vi "Get Sub Object.vi"(8 "error in":errorcluster, 9 "Sub Index":u8 format="%02x", 10 "Index":u16 format="%04x", 11 "Obj Dict in":refnum<class "Object Dictionary.lvclass">) -> (0 "error out":errorcluster, 2 "Sub Obj":refnum<class "Sub Object.lvclass">, 3 "Obj Dict out":refnum<class "Object Dictionary.lvclass">)   [LabVIEW 2020, in "CANopen.lvlib" / "Object Dictionary.lvclass"]
uses:
  Object Dictionary.lvclass
  Sub Object/Sub Object.lvclass
  Object Entry/Object Entry.lvclass
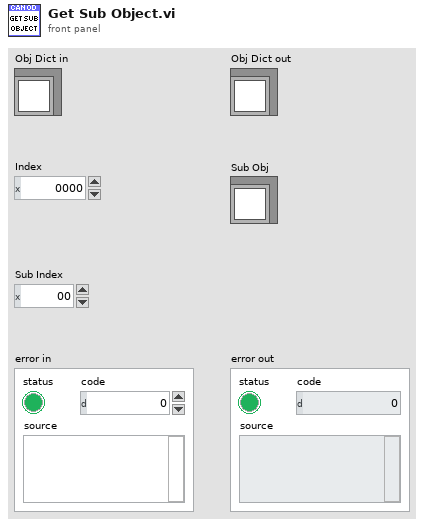
[diagram p1: front panel]
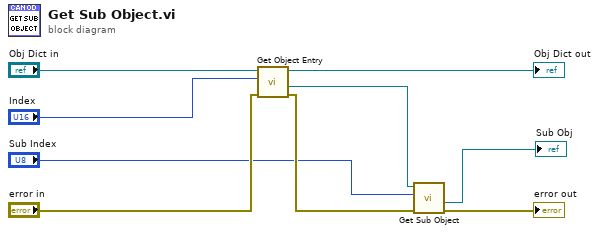
[diagram p0: block diagram]
diagram:
  n1 = call "Get Object Entry.vi"("error in"="error in", "OD Index"="Index", "Obj Dict in"="Obj Dict in") -> ("error out"=w3:errorcluster, "Obj Entry"=w2:refnum<class "Object Entry.lvclass">, "Obj Dict out"=→"Obj Dict out":refnum<class "Object Dictionary.lvclass">)  [unwired: 6 in]
  n2 = call "Get Sub Object.vi"("error in"=w3, "Sub Index"="Sub Index", "Obj Entry in"=w2) -> ("error out"=→"error out":errorcluster, "Sub Object"=→"Sub Obj":refnum<class "Sub Object.lvclass">)  [unwired: 6 in, 1 out]
